vi "New Parameter Message.vi"(8 "error in (no error)":errorcluster, 10 "New parameter":variant, 11 "Temperature Controller in":refnum<class "Temperature Controller.lvclass">) -> (0 "error out":errorcluster, 2 "New Parameter Message":T1, 3 "Temperature Controller out":refnum<class "Temperature Controller.lvclass">)   [LabVIEW 2020, in "Temperature Controller.lvclass"]
doc: "Dynamic dispatch for each child controller type to provide it's proper message for setting a new parameter value (setpoint)."
uses:
  Temperature Controller.lvclass
  <userlib>/RxnRover/DynamicReentrant/src/Type Defs/Message.ctl
  <userlib>/RxnRover/DynamicReentrant/Dynamic Reentrant.lvlib
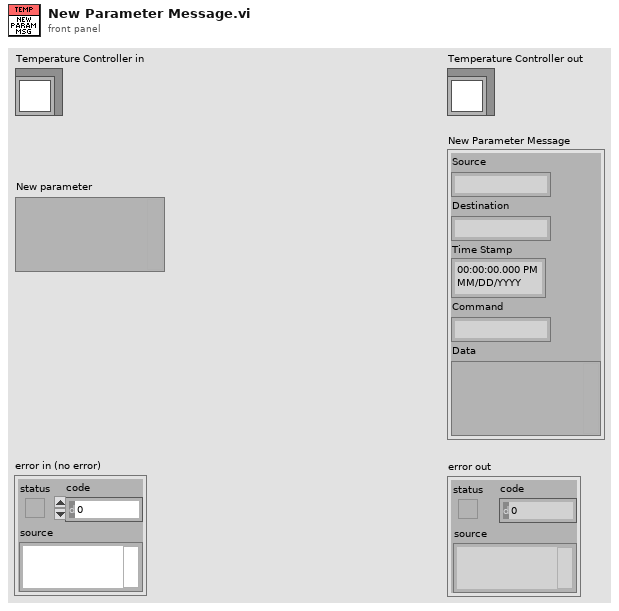
[diagram p1: front panel]
types:
  T1 = typedef "Dynamic Reentrant.lvlib/Message.ctl" = cluster{"Source":string, "Destination":string, "Time Stamp":timestamp, "Command":string, "Data":variant}
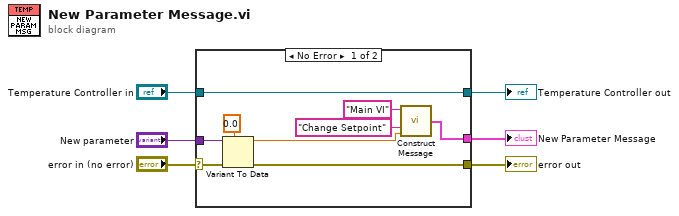
[diagram p0: block diagram]
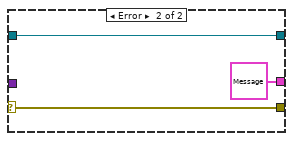
[diagram p2: hidden frame]
diagram:
  n1 = case shown="No Error" "error in (no error)" {
    selector: "error in (no error)" -> [w8 w17]
    tunnel: "New parameter" -> [w15 _]
    tunnel: [w12 T1 {"Source"="", "Destination"="", "Time Stamp"=timestamp(0 s since 1904-01-01), "Command"="", "Data"=variant} ("output cluster")] -> w5
    tunnel: [w11 w17] -> w4
    tunnel: "Temperature Controller in" -> [w7 w16]
    tunnel: [w7 w16] -> w1
    frame No Error {
      n2 = Variant To Data(error in=w8, type=0.0, Variant=w15) -> (data=w13:dbl, error out=w11:errorcluster)
      n3 = call <userlib>:"Construct Message.vi"("Data"=w13, "Command"="Change Setpoint", "Source"="Main VI") -> ("Message Cluster"=w12:T1)  [unwired: 3 in]
    }
    frame Error {
    }
  }
  "error out" <- w4
  "Temperature Controller out" <- w1
  "New Parameter Message" <- w5
